vi "Length_Message_Boatloader.vi"(5 "string":string="04 03", 11 "error in":errorcluster) -> (6 "hex integer string":string, 8 "Message":string="04 03", 15 "error out":errorcluster)   [LabVIEW 2023]
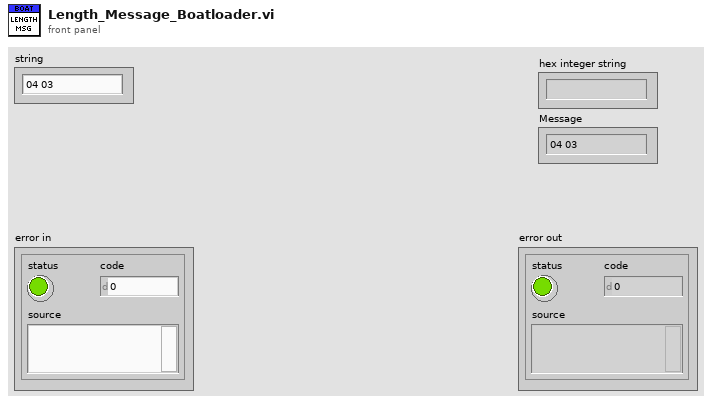
[diagram p1: front panel]
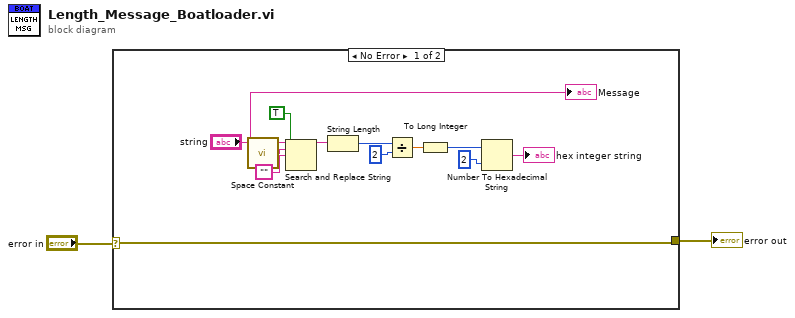
[diagram p0: block diagram]
diagram:
  n1 = case shown="No Error" "error in" {
    selector: "error in" -> [w3 w15]
    tunnel: [w3 w15] -> w2
    frame No Error {
      n2 = call <vilib>:"Space Constant.vi"() -> ("String"=w12:string)
      n3 = Search and Replace String(replace all?=TRUE ("replace all? (F)"), input string="string", search string=w12, replace string="") -> (result string=w10:string)  [unwired: 4 in, 3 out]
      n4 = String Length(string=w10) -> (length=w7:i32)
      n5 = Divide(x=w7, y=2) -> (x/y=w5:dbl)
      n6 = To Long Integer(number=w5) -> (32bit integer=w4:i32)
      n7 = Number To Hexadecimal String(1:i16 2 ("width (-)"), 2:w4) -> (0:→"hex integer string":string)
      "Message" <- "string"
    }
    frame Error {
    }
  }
  "error out" <- w2
